vi "SSE Example Main.vi"() -> ()   [LabVIEW 2020, in "Server Sent Events Example.lvlib"]
uses:
  Server Sent Events Example.lvlib
  lv-http-server/HTTP Server/SSE Client/SSE Client.lvclass
  SSEHomeController/SSEHomeController.lvclass
  C:/dev/lv20CE/relink/lv-http-server/HTTP Server/Handler/Handler.lvclass
  SSE Manager/SSE Manager.lvclass
  C:/dev/lv20CE/relink/lv-http-server/HTTP Server/SSE Manager/SSE Manager.lvclass
  lv-http-server/HTTP Server/Server/Add Connection Handler.vi
  lv-http-server/HTTP Server/Server/Add Request Handler.vi
  lv-http-server/HTTP Server/Server/Add Route Handler.vi
  lv-http-server/HTTP Server/Server/Add Controller Handler.vi
  lv-http-server/HTTP Server/Server/Add Controller.vi
  lv-http-server/HTTP Server/Server/Add Response Handler.vi
  lv-http-server/HTTP Server/Server/Add Complete Handler.vi
  lv-http-server/HTTP Server/Server/Add Exception Handler.vi
  lv-http-server/HTTP Server/Connection Handler/Connection Handler.lvclass
  lv-http-server/HTTP Server/Request Handler/Request Handler.lvclass
  lv-http-server/HTTP Server/Route Handler/Route Handler.lvclass
  lv-http-server/HTTP Server/Controller Handler/Controller Handler.lvclass
  lv-http-server/HTTP Server/Controller/Controller.lvclass
  lv-http-server/HTTP Server/Response Handler/Response Handler.lvclass
  lv-http-server/HTTP Server/Complete Handler/Complete Handler.lvclass
  lv-http-server/HTTP Server/Exception Handler/Exception Handler.lvclass
  lv-http-server/HTTP Server/Handler/Handler.lvclass
  lv-http-server/HTTP Server/Server/Server.lvclass
  lv-web-crypto/lv-json/JSON/JSON.lvlib
panel:
  out "Last Data":string
  out "# Clients":i32
  # "Click X to stop example."
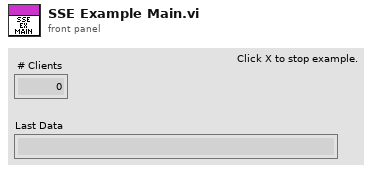
[diagram p1: front panel]
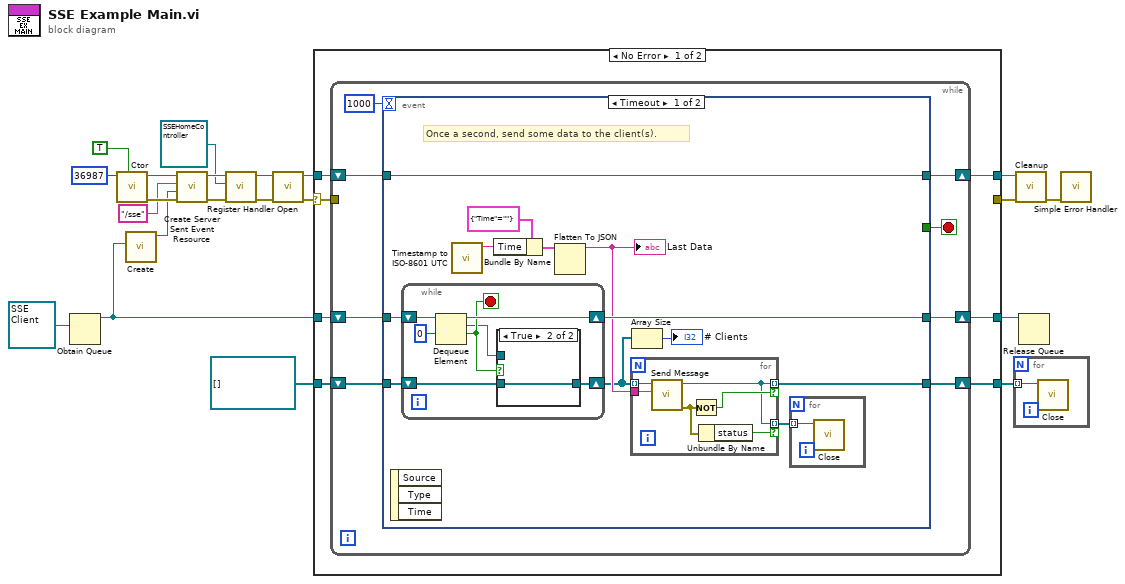
[diagram p0: block diagram]
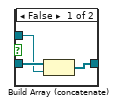
[diagram p2: hidden frame]
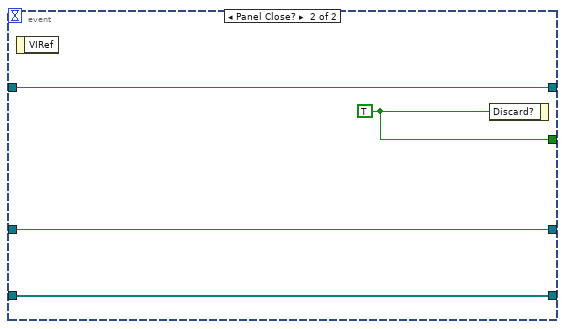
[diagram p3: hidden frame]
diagram:
  n1 = Obtain Queue(element data type=refnum<class "SSE Client.lvclass"> refnum ("HTTP Server:SSE Client.lvclass")) -> (queue out=w9:refnum<queue>)  [unwired: 4 in, 2 out]
  n2 = call "Ctor.vi"("Debug (F)"=TRUE, "HTTP Port (80)"=u16 36987 ("Port (8080)")) -> ("error out"=w21:errorcluster, "Server out"=w17:refnum<class "Server.lvclass">)  [unwired: 8 in]
  n3 = call "Create.vi"("New Client Q"=w9) -> ("SSE Manager out"=w15:refnum<class "SSE Manager.lvclass">)  [unwired: 9 in, 1 out]
  n4 = call "Create Server Sent Event Resource.vi"("error in (no error)"=w21, "SSE Manager"=w15, "Path"="/sse", "Server in"=w17) -> ("error out"=w13:errorcluster, "Server out"=w14:refnum<class "Server.lvclass">)  [unwired: 6 in]
  n5 = call "Register Handler.vi"("error in (no error)"=w13, "Handler"=refnum<class "SSEHomeController.lvclass"> refnum ("Server Sent Events Example.lvlib:SSEHomeController.lvclass"), "Server in"=w14) -> ("error out"=w10:errorcluster, "Server out"=w11:refnum<class "Server.lvclass">)  [unwired: 7 in]
  n6 = call "Open.vi"("error in (no error)"=w10, "Server in"=w11) -> ("error out"=w7:errorcluster, "Server out"=w8:refnum<class "Server.lvclass">)  [unwired: 8 in]
  n7 = case shown="No Error" w7 {
    selector: w7 -> [w26 w73]
    tunnel: w9 -> [w28 w71]
    tunnel: w8 -> [w27 w72]
    tunnel: [_ w73] -> w5
    tunnel: [w25 w72] -> w6
    tunnel: [w24 w71] -> w3
    tunnel: refnum<class "SSE Client.lvclass">[] [] -> [w23 _]
    tunnel: [w22 _] -> w1
    frame No Error {
      n8 = while {
        tunnel: w26 -> [_]
        shift-right: [w33] -> w25
        shift-left: w27 -> [w34]
        shift-right: [w32] -> w24
        shift-left: w28 -> [w35]
        shift-right: [w29] -> w22
        shift-left: w23 -> [w30]
        stop <- w31 stop-if-true
        n9 = event shown="[0] Timeout" {
          selector: _ -> [_ _]
          dyn-events: _ -> [_ _]
          timeout: 1000 -> [_ _]
          tunnel: w35 -> [w47 w69]
          tunnel: w34 -> [w48 w70]
          tunnel: [w48 w70] -> w33
          tunnel: [w42 w69] -> w32
          tunnel: [_ w68] -> w31
          tunnel: w30 -> [w46 w67]
          tunnel: [w41 w67] -> w29
          event Timeout {
            # "Once a second, send some data to the client(s)."
            n10 = event-data() -> ()  [unwired: 1 in, 3 out]
            n11 = while {
              shift-right: [w60] -> w42
              shift-left: w47 -> [w62]
              shift-right: [w56] -> w39
              shift-left: w46 -> [w58]
              stop <- w59 stop-if-true
              n12 = Dequeue Element(queue=w62, timeout in ms (-1)=0) -> (queue out=w60:refnum<queue>, element=w57:refnum<class "SSE Client.lvclass">, timed out?=w59:bool)  [unwired: 1 in, 1 out]
              n13 = case shown="True" w59 {
                tunnel: w58 -> [w65 w66]
                tunnel: w57 -> [w64 _]
                tunnel: [w63 w66] -> w56
                frame False {
                  n14 = Build Array (concatenate)(w65, w64) -> (w63:refnum<class "SSE Client.lvclass">[])
                }
                frame True {
                }
              }
            }
            n15 = call "Timestamp to ISO-8601 UTC.vi"() -> ("ISO 8601 UTC"=w44:string)  [unwired: 11 in]
            n16 = Bundle By Name(cluster=cluster{"Time":string} {"Time"=""}, "Time"=w44) -> (w43:cluster{"Time":string})
            n17 = Flatten To JSON(anything=w43) -> (JSON string=w40:string)  [unwired: 2 in, 1 out]
            "Last Data" <- w40
            n18 = for {
              tunnel: w39 -> [w55] mode=indexing
              tunnel: [w52] -> w41 mode=indexing if=w54
              tunnel: w40 -> [w53]
              tunnel: [w52] -> w37 mode=indexing if=w50
              n19 = call "Send Message.vi"("Data"=w53, "SSE Client in"=w55) -> ("error out"=w51:errorcluster, "SSE Client out"=w52:refnum<class "SSE Client.lvclass">)  [unwired: 8 in]
              n20 = Not(x=w51) -> (.not. x?=w54:bool)
              n21 = Unbundle By Name(w51) -> ("status"=w50:bool)
            }
            n22 = Array Size(array=w39) -> (size(s)=→"# Clients":i32)
            n23 = for {
              tunnel: w37 -> [w49] mode=indexing
              n24 = call "Close.vi"("SSE Client in"=w49) -> ()  [unwired: 10 in, 1 out]
            }
          }
          event Panel Close? {
            w68 = TRUE ("Discard?")
            n25 = event-data() -> ()  [unwired: 1 in, 1 out]
            n26 = event-data("Discard?"=w68) -> ()  [unwired: 1 in, 1 out]
          }
        }
      }
    }
    frame Error {
    }
  }
  n27 = for {
    tunnel: w1 -> [w74] mode=indexing
    n28 = call "Close.vi"("SSE Client in"=w74) -> ()  [unwired: 10 in, 1 out]
  }
  n29 = call "Cleanup.vi"("error in (no error)"=w5, "Server in"=w6) -> ("error out"=w4:errorcluster)  [unwired: 9 in]
  n30 = Release Queue(queue=w3) -> ()  [unwired: 2 in, 3 out]
  n31 = call <vilib>:"Simple Error Handler.vi"("error in (no error)"=w4) -> ()  [unwired: 4 in, 5 out]
